vi "PID_controller_13.vi"() -> ()   [LabVIEW 2011]
uses:
  <vilib>/Analysis/NI_AALPro.lvlib
panel:
  out "P(t)":cluster{dbl, "Value":dbl}[](array[cluster])
  in  "Fitting points":i32
  in  "stop":bool
  out "fit":cluster{"element":dbl, "Value":dbl}[](array[cluster])
  out "err_avg":dbl
  out "Setpoint":string
  out "Angle (deg)":string
  in  "Ks":dbl
  out "dt(s)":dbl
  out "windup error":dbl
  out "tPrev":dbl
  out "target value":dbl
  out "error(t-t0)":cluster{dbl, "Value":dbl}[](array[cluster])
  out "error":dbl
  out "tStart(s)":dbl
  out "S00":dbl
  out "S10":dbl
  out "S20":dbl
  out "S11":dbl
  out "S01":dbl
  out "weight":dbl[](array[numeric])
  in  "# of points to watch":i32
  in  "tSmooth(s)":dbl=-1.0
  out "t0":dbl
  out "error(t)":cluster{dbl, "Value":dbl}[](array[cluster])
  out "error out":errorcluster
  out "first":bool=TRUE
  out "P (torr)":string
  out "XY Graph":T1(graph)
  out "current value":dbl
  in  "Period (s)":dbl
  out "dValue":dbl
  out "derivative":dbl
  out "integral":dbl
  out "Current angle (deg)":dbl
  in  "Kd":dbl
  in  "Ki":dbl
  in  "Kp":dbl
  out "Current P (torr)":dbl
  in  "Set Point (torr)":dbl
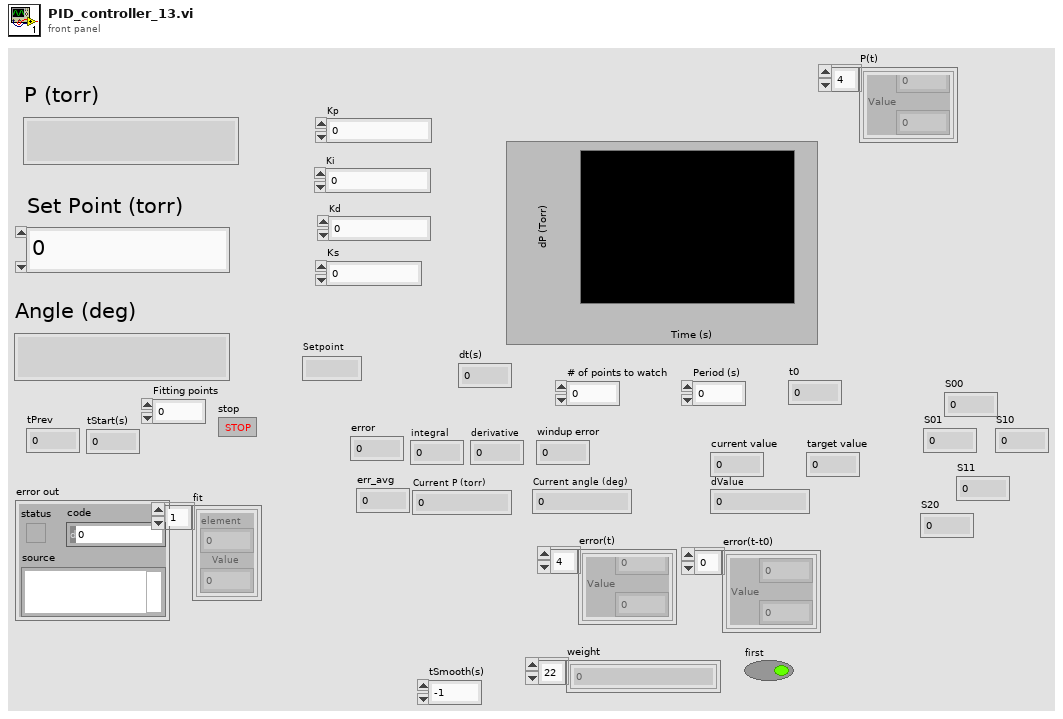
[diagram p1: front panel]
types:
  T1 = cluster{"Value":cluster{"element":dbl, "Value":dbl}[]}[]
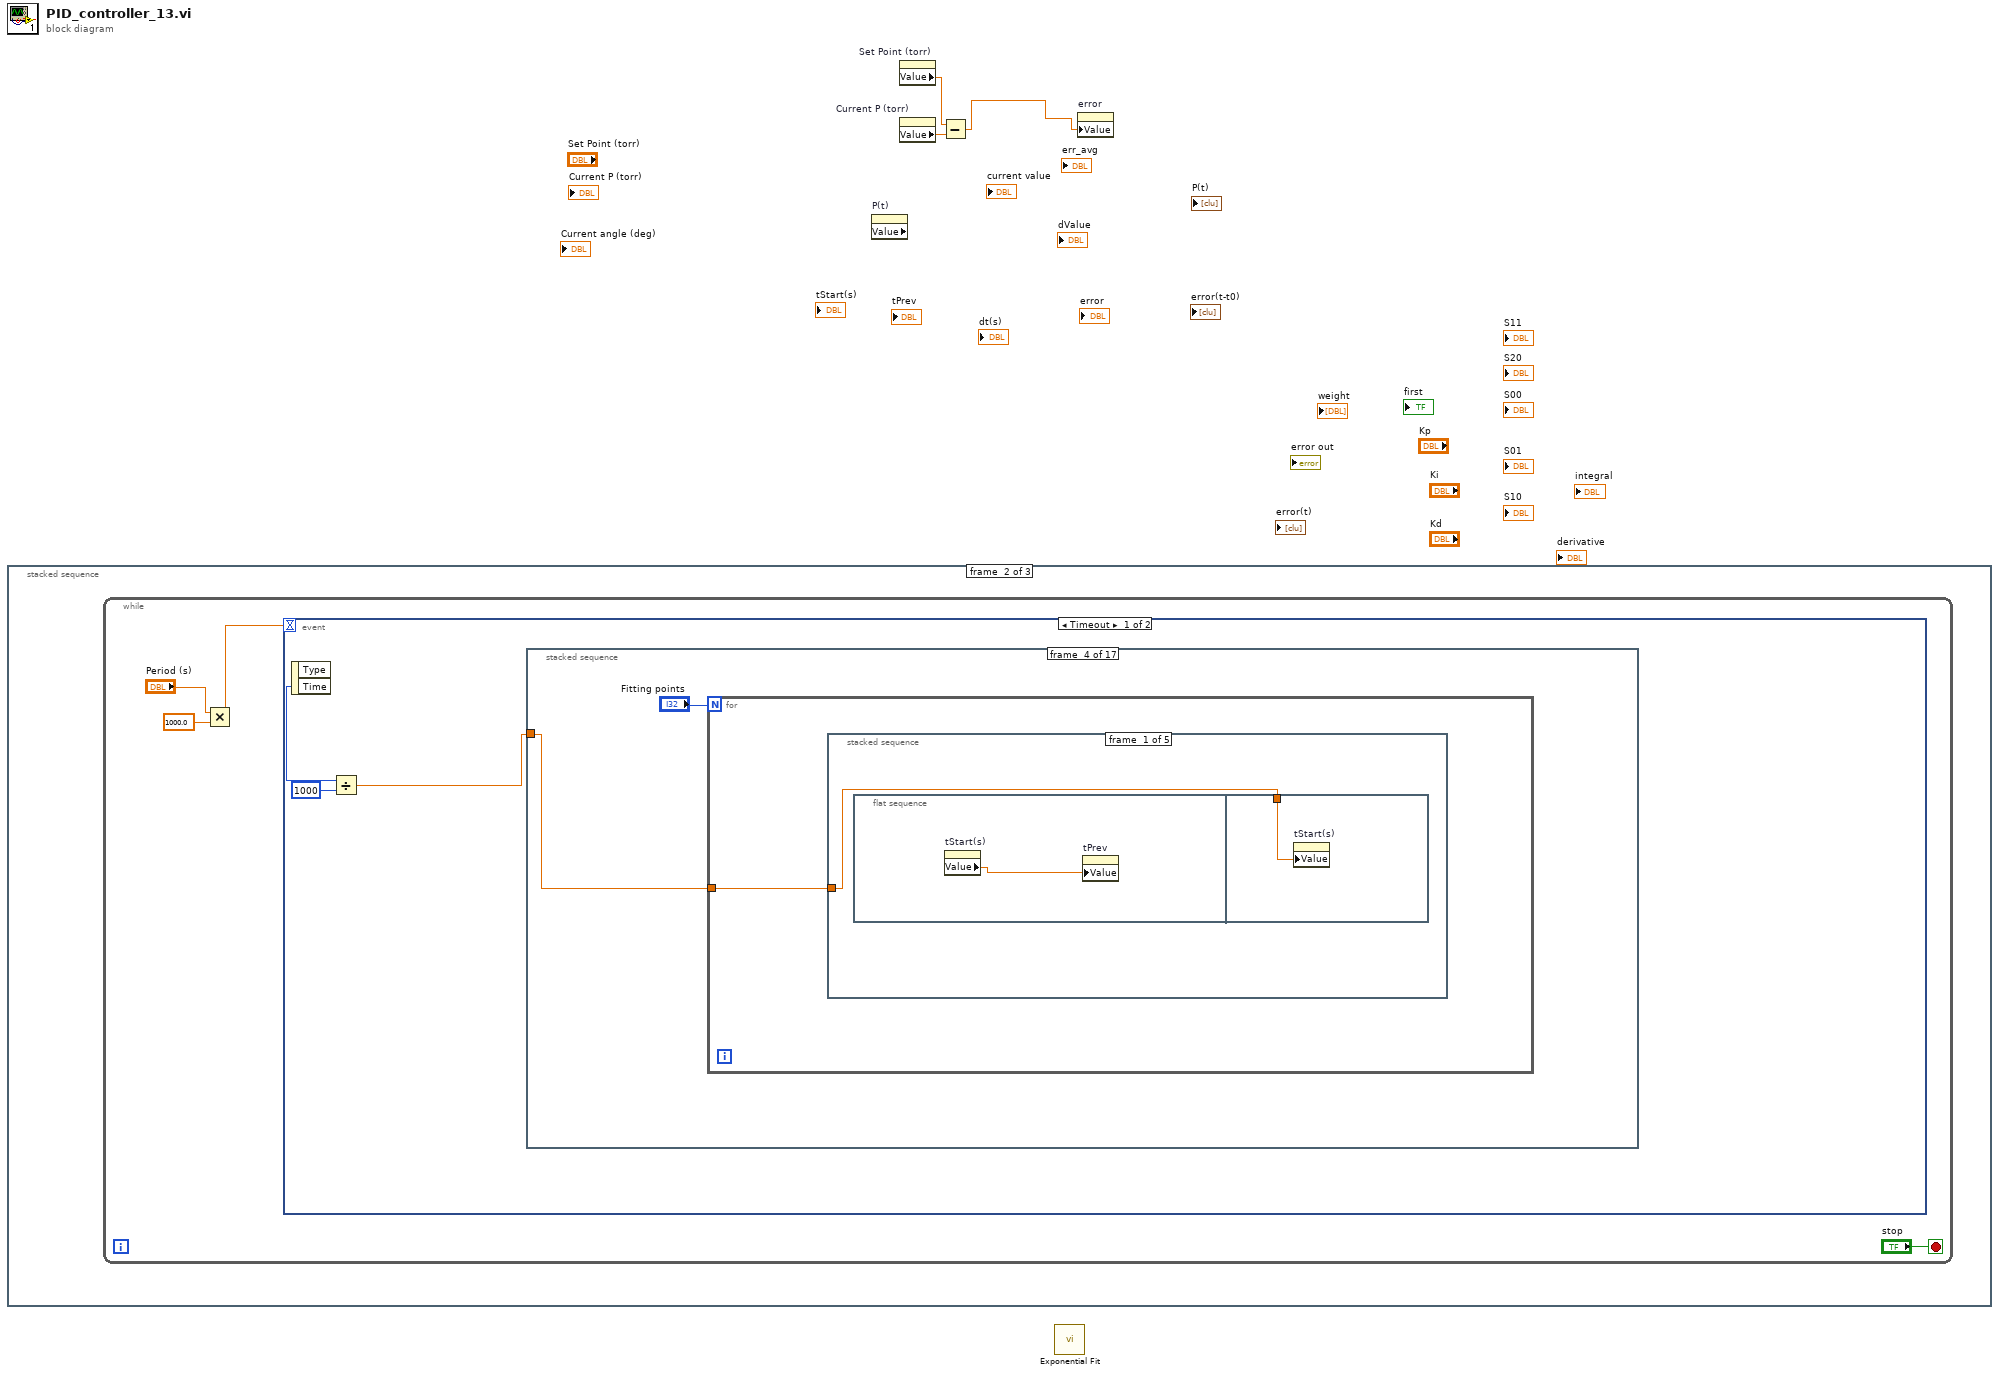
[diagram p0: block diagram]
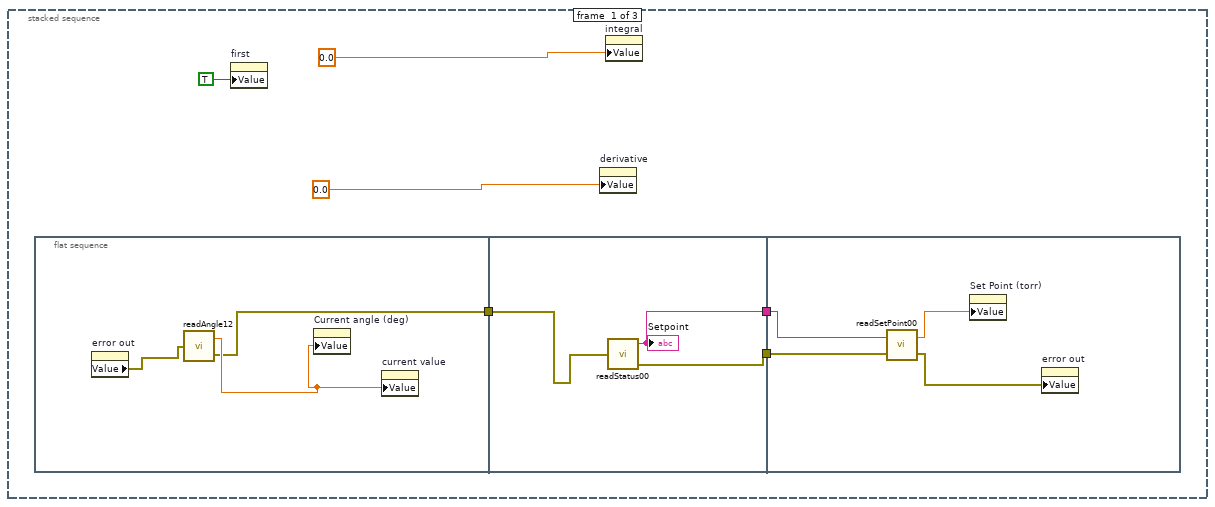
[diagram p2: hidden frame]
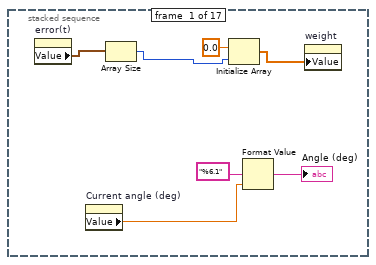
[diagram p3: hidden frame]
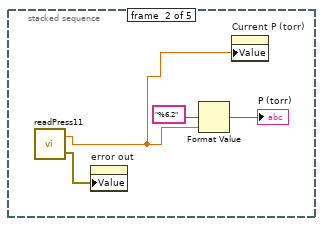
[diagram p6: hidden frame]
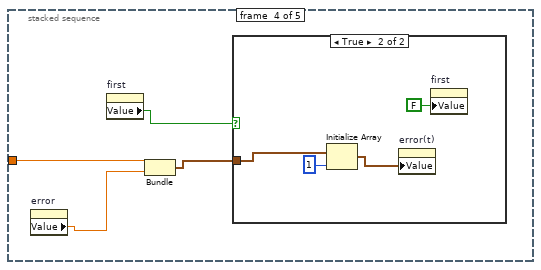
[diagram p8: hidden frame]
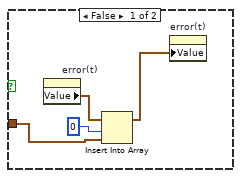
[diagram p9: hidden frame]
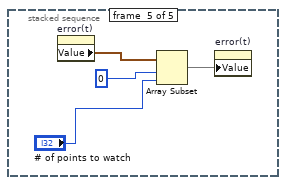
[diagram p10: hidden frame]
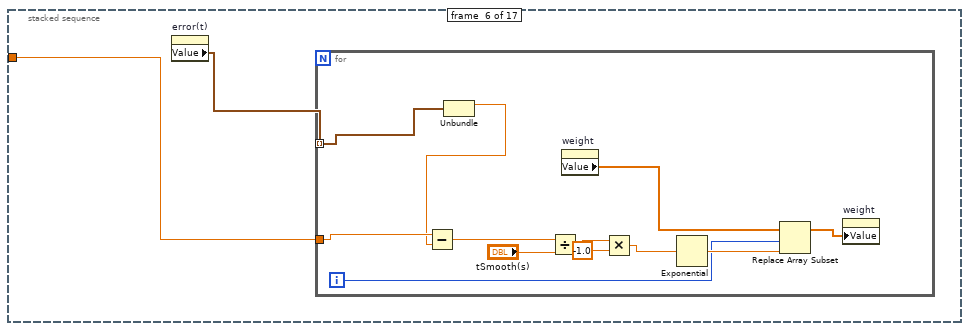
[diagram p12: hidden frame]
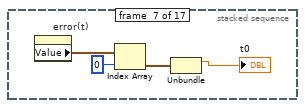
[diagram p13: hidden frame]
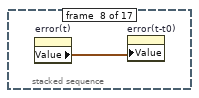
[diagram p14: hidden frame]
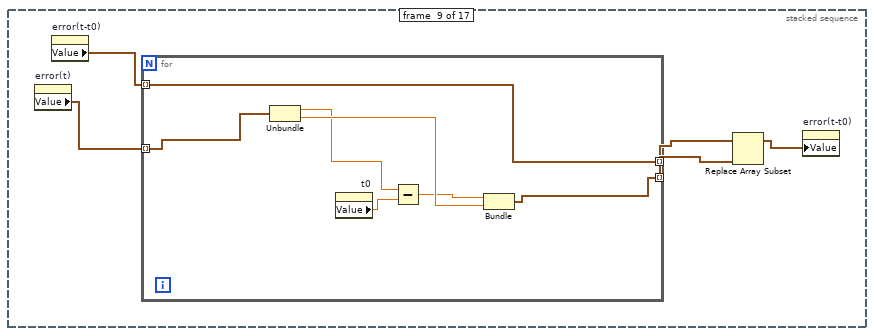
[diagram p15: hidden frame]
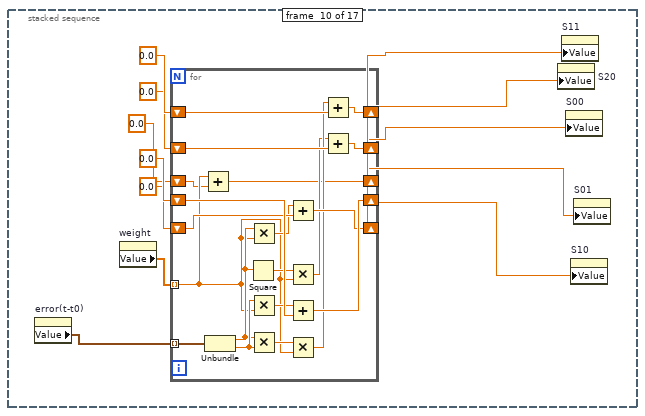
[diagram p16: hidden frame]
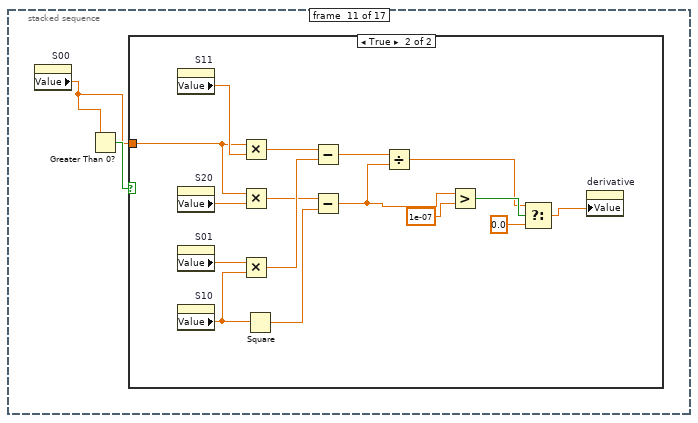
[diagram p17: hidden frame]
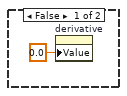
[diagram p18: hidden frame]
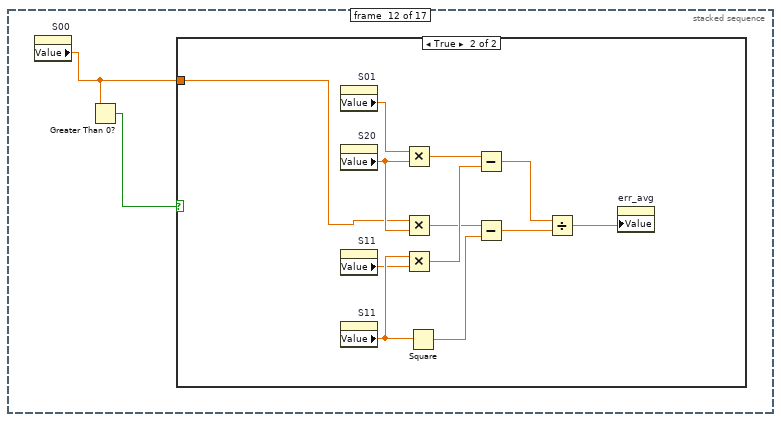
[diagram p19: hidden frame]
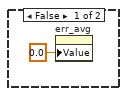
[diagram p20: hidden frame]
diagram:
  n1 = stacked-sequence {
    frame #0 {
      n2 = flat-sequence {
        tunnel: [w10] -> w4
        tunnel: [w15] -> w6
        tunnel: [w14] -> w5
        tunnel: w4 -> [w13]
        tunnel: w6 -> [w19]
        tunnel: w5 -> [w18]
        frame #0 {
          n3 = property on="error out" class="Clust (strict)"() -> ("Value"=w12:errorcluster)  [unwired: 2 in, 2 out]
          n4 = call "readAngle12.vi"("error in"=w12) -> ("angle"=w11:dbl, "error out"=w10:errorcluster)
          n5 = property on="Current angle (deg)" class="DigNum (strict)"("Value"=w11) -> ()  [unwired: 2 in, 2 out]
          n6 = property on="current value" class="DigNum (strict)"("Value"=w11) -> ()  [unwired: 2 in, 2 out]
        }
        frame #1 {
          n7 = call "readStatus00.vi"("error in"=w13) -> ("Setpoint"=w15:string, "error out"=w14:errorcluster)  [unwired: 1 out]
          "Setpoint" <- w15
        }
        frame #2 {
          n8 = call "readSetPoint00.vi"("error in"=w18, "Setpoint"=w19) -> ("error out"=w17:errorcluster, "P"=w16:dbl)
          n9 = property on="Set Point (torr)" class="DigNum (strict)"("Value"=w16) -> ()  [unwired: 2 in, 2 out]
          n10 = property on="error out" class="Clust (strict)"("Value"=w17) -> ()  [unwired: 2 in, 2 out]
        }
      }
      n11 = property on="first" class="Bool (strict)"("Value"=TRUE ("first")) -> ()  [unwired: 2 in, 2 out]
      n12 = property on="derivative" class="DigNum (strict)"("Value"=0.0 ("derivative")) -> ()  [unwired: 2 in, 2 out]
      n13 = property on="integral" class="DigNum (strict)"("Value"=0.0 ("integral")) -> ()  [unwired: 2 in, 2 out]
    }
    frame #1 {
      n14 = while {
        stop <- "stop" stop-if-true
        n15 = Multiply(x="Period (s)", y=1000.0) -> (x*y=w21:dbl)
        n16 = event shown="[0] Timeout" {
          selector: _ -> [_ _]
          dyn-events: _ -> [_ _]
          timeout: w21 -> [_ _]
          event Timeout {
            n17 = event-data() -> ("Time"=w26:u32)  [unwired: 1 in, 1 out]
            n18 = Divide(x=w26, y=u32 1000) -> (x/y=w24:dbl)
            n19 = stacked-sequence {
              tunnel: w24 -> [_ _ w34 w35 _ w61 _ _ _ _ _ _ _ _ _ _ _]
              frame #0 {
                n20 = property on="error(t)" class="Arr (strict)"() -> ("Value"=w30:cluster{dbl, "Value":dbl}[])  [unwired: 2 in, 2 out]
                n21 = property on="Current angle (deg)" class="DigNum (strict)"() -> ("Value"=w31:dbl)  [unwired: 2 in, 2 out]
                n22 = Array Size(array=w30) -> (size(s)=w28:i32)
                n23 = Initialize Array(0.0 ("element"), w28) -> (w27:dbl[])
                n24 = Format Value(format string="%6.1", value (0)=w31) -> (output string=→"Angle (deg)":string)  [unwired: 1 in]
                n25 = property on="weight" class="Arr (strict)"("Value"=w27) -> ()  [unwired: 2 in, 2 out]
              }
              frame #1 {
              }
              frame #2 {
                n26 = stacked-sequence {
                  tunnel: w34 -> [_]
                  frame #0 {
                  }
                }
              }
              frame #3 {
                n27 = for {
                  N: "Fitting points" -> [_]
                  tunnel: w35 -> [w37]
                  n28 = stacked-sequence {
                    tunnel: w37 -> [w38 _ _ w47 _]
                    frame #0 {
                      n29 = flat-sequence {
                        tunnel: w38 -> [w40]
                        frame #0 {
                          n30 = property on="tStart(s)" class="DigNum (strict)"() -> ("Value"=w39:dbl)  [unwired: 2 in, 2 out]
                          n31 = property on="tPrev" class="DigNum (strict)"("Value"=w39) -> ()  [unwired: 2 in, 2 out]
                        }
                        frame #1 {
                          n32 = property on="tStart(s)" class="DigNum (strict)"("Value"=w40) -> ()  [unwired: 2 in, 2 out]
                        }
                      }
                    }
                    frame #1 {
                      n33 = call "readPress11.vi"() -> ("P"=w42:dbl, "error out"=w41:errorcluster)  [unwired: 1 in]
                      n34 = property on="error out" class="Clust (strict)"("Value"=w41) -> ()  [unwired: 2 in, 2 out]
                      n35 = Format Value(format string="%6.2", value (0)=w42) -> (output string=→"P (torr)":string)  [unwired: 1 in]
                      n36 = property on="Current P (torr)" class="DigNum (strict)"("Value"=w42) -> ()  [unwired: 2 in, 2 out]
                    }
                    frame #2 {
                    }
                    frame #3 {
                      n37 = property on="error" class="DigNum (strict)"() -> ("Value"=w45:dbl)  [unwired: 2 in, 2 out]
                      n38 = property on="first" class="Bool (strict)"() -> ("Value"=w48:bool)  [unwired: 2 in, 2 out]
                      n39 = Bundle(w47, "Value"=w45) -> (w46:cluster{dbl, "Value":dbl})  [unwired: 1 in]
                      n40 = case shown="True" w48 {
                        tunnel: w46 -> [w50 w55]
                        frame False {
                          n41 = property on="error(t)" class="Arr (strict)"() -> ("Value"=w51:cluster{dbl, "Value":dbl}[])  [unwired: 2 in, 2 out]
                          n42 = Insert Into Array(array=w51, index=0, new element=w50) -> (w49:cluster{dbl, "Value":dbl}[])
                          n43 = property on="error(t)" class="Arr (strict)"("Value"=w49) -> ()  [unwired: 2 in, 2 out]
                        }
                        frame True {
                          n44 = Initialize Array(w55, 1 ("dimension size")) -> (w53:cluster{dbl, "Value":dbl}[])
                          n45 = property on="error(t)" class="Arr (strict)"("Value"=w53) -> ()  [unwired: 2 in, 2 out]
                          n46 = property on="first" class="Bool (strict)"("Value"=FALSE ("first")) -> ()  [unwired: 2 in, 2 out]
                        }
                      }
                    }
                    frame #4 {
                      n47 = property on="error(t)" class="Arr (strict)"() -> ("Value"=w58:cluster{dbl, "Value":dbl}[])  [unwired: 2 in, 2 out]
                      n48 = Array Subset(array=w58, index=0, length="# of points to watch") -> (w60:cluster{dbl, "Value":dbl}[])
                      n49 = property on="error(t)" class="Arr (strict)"("Value"=w60) -> ()  [unwired: 2 in, 2 out]
                    }
                  }
                }
              }
              frame #4 {
              }
              frame #5 {
                n50 = property on="error(t)" class="Arr (strict)"() -> ("Value"=w62:cluster{dbl, "Value":dbl}[])  [unwired: 2 in, 2 out]
                n51 = for {
                  tunnel: w62 -> [w74] mode=indexing
                  tunnel: w61 -> [w73]
                  i -> [w69]
                  n52 = Unbundle(w74) -> (w72:dbl)  [unwired: 1 out]
                  n53 = Subtract(x=w73, y=w72) -> (x-y=w67:dbl)
                  n54 = Divide(x=w67, y="tSmooth(s)") -> (x/y=w65:dbl)
                  n55 = property on="weight" class="Arr (strict)"() -> ("Value"=w70:dbl[])  [unwired: 2 in, 2 out]
                  n56 = Multiply(x=w65, y=-1.0) -> (x*y=w63:dbl)
                  n57 = Exponential(1:w63) -> (0:w71:dbl)
                  n58 = Replace Array Subset(array=w70, new element=w71, index=w69) -> (w68:dbl[])
                  n59 = property on="weight" class="Arr (strict)"("Value"=w68) -> ()  [unwired: 2 in, 2 out]
                }
              }
              frame #6 {
                n60 = property on="error(t)" class="Arr (strict)"() -> ("Value"=w78:cluster{dbl, "Value":dbl}[])  [unwired: 2 in, 2 out]
                n61 = Index Array(array=w78, index=0) -> (element=w76:cluster{dbl, "Value":dbl})
                n62 = Unbundle(w76) -> (→"t0":dbl)  [unwired: 1 out]
              }
              frame #7 {
                n63 = property on="error(t)" class="Arr (strict)"() -> ("Value"=w79:cluster{dbl, "Value":dbl}[])  [unwired: 2 in, 2 out]
                n64 = property on="error(t-t0)" class="Arr (strict)"("Value"=w79) -> ()  [unwired: 2 in, 2 out]
              }
              frame #8 {
                n65 = property on="error(t)" class="Arr (strict)"() -> ("Value"=w84:cluster{dbl, "Value":dbl}[])  [unwired: 2 in, 2 out]
                n66 = property on="error(t-t0)" class="Arr (strict)"() -> ("Value"=w82:cluster{dbl, "Value":dbl}[])  [unwired: 2 in, 2 out]
                n67 = for {
                  tunnel: w84 -> [w87] mode=indexing
                  tunnel: [w86] -> w83 mode=indexing
                  tunnel: w82 -> [w85] mode=indexing
                  tunnel: [w85] -> w81 mode=indexing
                  n68 = Unbundle(w87) -> (w88:dbl, "Value"=w90:dbl)
                  n69 = property on="t0" class="DigNum (strict)"() -> ("Value"=w91:dbl)  [unwired: 2 in, 2 out]
                  n70 = Subtract(x=w88, y=w91) -> (x-y=w89:dbl)
                  n71 = Bundle(w89, "Value"=w90) -> (w86:cluster{dbl, "Value":dbl})  [unwired: 1 in]
                }
                n72 = Replace Array Subset(array=w81, new element=w83) -> (w80:cluster{dbl, "Value":dbl}[])  [unwired: 1 in]
                n73 = property on="error(t-t0)" class="Arr (strict)"("Value"=w80) -> ()  [unwired: 2 in, 2 out]
              }
              frame #9 {
                n74 = property on="error(t-t0)" class="Arr (strict)"() -> ("Value"=w92:cluster{dbl, "Value":dbl}[])  [unwired: 2 in, 2 out]
                n75 = property on="weight" class="Arr (strict)"() -> ("Value"=w99:dbl[])  [unwired: 2 in, 2 out]
                n76 = for {
                  tunnel: w92 -> [w119] mode=indexing
                  shift-right: [w120] -> w94
                  shift-left: 0.0 -> [w123]
                  shift-right: [w116] -> w97
                  shift-left: 0.0 -> [w122]
                  shift-right: [w115] -> w96
                  shift-left: 0.0 -> [w121]
                  shift-right: [w117] -> w93
                  shift-left: 0.0 -> [w118]
                  tunnel: w99 -> [w106] mode=indexing
                  shift-right: [w104] -> w95
                  shift-left: 0.0 -> [w105]
                  n77 = Add(x=w106, y=w105) -> (x+y=w104:dbl)
                  n78 = Unbundle(w119) -> (w108:dbl, "Value"=w114:dbl)
                  n79 = Square(x=w108) -> (x^2=w110:dbl)
                  n80 = Multiply(x=w108, y=w106) -> (x*y=w107:dbl)
                  n81 = Multiply(x=w114, y=w106) -> (x*y=w113:dbl)
                  n82 = Multiply(x=w108, y=w114) -> (x*y=w112:dbl)
                  n83 = Add(x=w107, y=w118) -> (x+y=w117:dbl)
                  n84 = Multiply(x=w110, y=w106) -> (x*y=w109:dbl)
                  n85 = Add(x=w113, y=w123) -> (x+y=w120:dbl)
                  n86 = Multiply(x=w112, y=w106) -> (x*y=w111:dbl)
                  n87 = Add(x=w111, y=w122) -> (x+y=w116:dbl)
                  n88 = Add(x=w109, y=w121) -> (x+y=w115:dbl)
                }
                n89 = property on="S20" class="DigNum (strict)"("Value"=w96) -> ()  [unwired: 2 in, 2 out]
                n90 = property on="S11" class="DigNum (strict)"("Value"=w97) -> ()  [unwired: 2 in, 2 out]
                n91 = property on="S00" class="DigNum (strict)"("Value"=w95) -> ()  [unwired: 2 in, 2 out]
                n92 = property on="S10" class="DigNum (strict)"("Value"=w93) -> ()  [unwired: 2 in, 2 out]
                n93 = property on="S01" class="DigNum (strict)"("Value"=w94) -> ()  [unwired: 2 in, 2 out]
              }
              frame #10 {
                n94 = property on="S00" class="DigNum (strict)"() -> ("Value"=w124:dbl)  [unwired: 2 in, 2 out]
                n95 = Greater Than 0?(x=w124) -> (x > 0?=w125:bool)
                n96 = case shown="True" w125 {
                  tunnel: w124 -> [_ w134]
                  frame False {
                    n97 = property on="derivative" class="DigNum (strict)"("Value"=0.0 ("derivative")) -> ()  [unwired: 2 in, 2 out]
                  }
                  frame True {
                    n98 = property on="S11" class="DigNum (strict)"() -> ("Value"=w136:dbl)  [unwired: 2 in, 2 out]
                    n99 = property on="S20" class="DigNum (strict)"() -> ("Value"=w135:dbl)  [unwired: 2 in, 2 out]
                    n100 = property on="S01" class="DigNum (strict)"() -> ("Value"=w133:dbl)  [unwired: 2 in, 2 out]
                    n101 = property on="S10" class="DigNum (strict)"() -> ("Value"=w137:dbl)  [unwired: 2 in, 2 out]
                    n102 = Multiply(x=w134, y=w136) -> (x*y=w142:dbl)
                    n103 = Multiply(x=w134, y=w135) -> (x*y=w140:dbl)
                    n104 = Multiply(x=w133, y=w137) -> (x*y=w141:dbl)
                    n105 = Square(x=w137) -> (x^2=w139:dbl)
                    n106 = Subtract(x=w142, y=w141) -> (x-y=w138:dbl)
                    n107 = Subtract(x=w140, y=w139) -> (x-y=w132:dbl)
                    n108 = Divide(x=w138, y=w132) -> (x/y=w128:dbl)
                    n109 = Greater?(x=w132, y=1e-07) -> (0:w130:bool)
                    n110 = Select(t=w128, s=w130, f=0.0) -> (s? t:f=w129:dbl)
                    n111 = property on="derivative" class="DigNum (strict)"("Value"=w129) -> ()  [unwired: 2 in, 2 out]
                  }
                }
              }
              frame #11 {
                n112 = property on="S00" class="DigNum (strict)"() -> ("Value"=w143:dbl)  [unwired: 2 in, 2 out]
                n113 = Greater Than 0?(x=w143) -> (x > 0?=w144:bool)
                n114 = case shown="True" w144 {
                  tunnel: w143 -> [_ w147]
                  frame False {
                    n115 = property on="err_avg" class="DigNum (strict)"("Value"=0.0 ("Pavg")) -> ()  [unwired: 2 in, 2 out]
                  }
                  frame True {
                    n116 = property on="S01" class="DigNum (strict)"() -> ("Value"=w148:dbl)  [unwired: 2 in, 2 out]
                    n117 = property on="S20" class="DigNum (strict)"() -> ("Value"=w151:dbl)  [unwired: 2 in, 2 out]
                    n118 = property on="S11" class="DigNum (strict)"() -> ("Value"=w149:dbl)  [unwired: 2 in, 2 out]
                    n119 = property on="S11" class="DigNum (strict)"() -> ("Value"=w150:dbl)  [unwired: 2 in, 2 out]
                    n120 = Multiply(x=w148, y=w151) -> (x*y=w156:dbl)
                    n121 = Multiply(x=w147, y=w151) -> (x*y=w153:dbl)
                    n122 = Multiply(x=w150, y=w149) -> (x*y=w157:dbl)
                    n123 = Square(x=w150) -> (x^2=w154:dbl)
                    n124 = Subtract(x=w156, y=w157) -> (x-y=w152:dbl)
                    n125 = Subtract(x=w153, y=w154) -> (x-y=w155:dbl)
                    n126 = Divide(x=w152, y=w155) -> (x/y=w146:dbl)
                    n127 = property on="err_avg" class="DigNum (strict)"("Value"=w146) -> ()  [unwired: 2 in, 2 out]
                  }
                }
              }
              frame #12 {
                n128 = property on="error(t-t0)" class="Arr (strict)"() -> ("Value"=w161:cluster{dbl, "Value":dbl}[])  [unwired: 2 in, 2 out]
                n129 = Array Size(array=w161) -> (size(s)=w160:i32)
                n130 = Greater?(x=w160, y=1) -> (0:w158:bool)
                n131 = case shown="True" w158 {
                  frame False {
                  }
                  frame True {
                    n132 = property on="error(t-t0)" class="Arr (strict)"() -> ("Value"=w165:cluster{dbl, "Value":dbl}[])  [unwired: 2 in, 2 out]
                    n133 = Array Size(array=w165) -> (size(s)=w175:i32)
                    n134 = Index Array(array=w165, index=0) -> (element=w173:cluster{dbl, "Value":dbl})
                    n135 = Unbundle(w173) -> (w168:dbl)  [unwired: 1 out]
                    n136 = Decrement(x=w175) -> (x-1=w174:i32)
                    n137 = Index Array(array=w165, index=w174) -> (element=w172:cluster{dbl, "Value":dbl})
                    n138 = Unbundle(w172) -> (w166:dbl)  [unwired: 1 out]
                    n139 = property on="derivative" class="DigNum (strict)"() -> ("Value"=w171:dbl)  [unwired: 2 in, 2 out]
                    n140 = property on="error" class="DigNum (strict)"() -> ("Value"=w169:dbl)  [unwired: 2 in, 2 out]
                    n141 = Multiply(x=w166, y=w171) -> (x*y=w170:dbl)
                    n142 = Add(x=w169, y=w170) -> (x+y=w167:dbl)
                    n143 = Bundle(w168, "Value"=w169) -> (w164:cluster{dbl, "Value":dbl})  [unwired: 1 in]
                    n144 = Bundle(w166, w167) -> (w163:cluster{dbl, dbl})  [unwired: 1 in]
                    n145 = Build Array(w164, w163) -> (→"fit":cluster{dbl, "Value":dbl}[])
                  }
                }
              }
              frame #13 {
                n146 = property on="error" class="DigNum (strict)"() -> ("Value"=w181:dbl)  [unwired: 2 in, 2 out]
                n147 = property on="tPrev" class="DigNum (strict)"() -> ("Value"=w182:dbl)  [unwired: 2 in, 2 out]
                n148 = property on="tStart(s)" class="DigNum (strict)"() -> ("Value"=w183:dbl)  [unwired: 2 in, 2 out]
                n149 = Subtract(x=w183, y=w182) -> (x-y=w177:dbl)
                n150 = property on="dt(s)" class="DigNum (strict)"("Value"=w177) -> ()  [unwired: 2 in, 2 out]
                n151 = property on="integral" class="DigNum (strict)"() -> ("Value"=w179:dbl)  [unwired: 2 in, 2 out]
                n152 = Multiply(x=w181, y=w177) -> (x*y=w180:dbl)
                n153 = Add(x=w180, y=w179) -> (x+y=w178:dbl)
                n154 = property on="integral" class="DigNum (strict)"("Value"=w178) -> ()  [unwired: 2 in, 2 out]
              }
              frame #14 {
                n155 = property on="error" class="DigNum (strict)"() -> ("Value"=w184:dbl)  [unwired: 2 in, 2 out]
                n156 = property on="Kp" class="DigNum (strict)"() -> ("Value"=w194:dbl)  [unwired: 2 in, 2 out]
                n157 = property on="integral" class="DigNum (strict)"() -> ("Value"=w192:dbl)  [unwired: 2 in, 2 out]
                n158 = property on="derivative" class="DigNum (strict)"() -> ("Value"=w190:dbl)  [unwired: 2 in, 2 out]
                n159 = property on="Ki" class="DigNum (strict)"() -> ("Value"=w193:dbl)  [unwired: 2 in, 2 out]
                n160 = property on="Kd" class="DigNum (strict)"() -> ("Value"=w191:dbl)  [unwired: 2 in, 2 out]
                n161 = Multiply(x=w191, y=w190) -> (x*y=w187:dbl)
                n162 = Multiply(x=w193, y=w192) -> (x*y=w188:dbl)
                n163 = Multiply(x=w194, y=w184) -> (x*y=w189:dbl)
                n164 = Add(x=w189, y=w188) -> (x+y=w186:dbl)
                n165 = Add(x=w186, y=w187) -> (x+y=w185:dbl)
                n166 = property on="dValue" class="DigNum (strict)"("Value"=w185) -> ()  [unwired: 2 in, 2 out]
              }
              frame #15 {
                w204 = 90.0 ("y")
                n167 = property on="dValue" class="DigNum (strict)"() -> ("Value"=w211:dbl)  [unwired: 2 in, 2 out]
                n168 = property on="current value" class="DigNum (strict)"() -> ("Value"=w212:dbl)  [unwired: 2 in, 2 out]
                n169 = Add(x=w212, y=w211) -> (x+y=w195:dbl)
                "target value" <- w195
                n170 = Less Than 0?(x=w195) -> (x < 0?=w208:bool)
                n171 = Select(t=0.0, s=w208, f=w195) -> (s? t:f=w205:dbl)
                n172 = property on="error out" class="Clust (strict)"() -> ("Value"=w210:errorcluster)  [unwired: 2 in, 2 out]
                n173 = Greater?(x=w205, y=w204) -> (0:w206:bool)
                n174 = Select(t=w204, s=w206, f=w205) -> (s? t:f=w196:dbl)
                n175 = Subtract(x=w196, y=w195) -> (x-y=w203:dbl)
                "windup error" <- w203
                n176 = call "setAngle_00.vi"("error in (no error)"=w210, "Angle (deg)"=w196) -> ("error out"=w209:errorcluster)
                n177 = property on="Current angle (deg)" class="DigNum (strict)"("Value"=w196) -> ()  [unwired: 2 in, 2 out]
                n178 = property on="dt(s)" class="DigNum (strict)"() -> ("Value"=w202:dbl)  [unwired: 2 in, 2 out]
                n179 = property on="current value" class="DigNum (strict)"("Value"=w196) -> ()  [unwired: 2 in, 2 out]
                n180 = property on="error out" class="Clust (strict)"("Value"=w209) -> ()  [unwired: 2 in, 2 out]
                n181 = Multiply(x=w203, y=w202) -> (x*y=w201:dbl)
                n182 = property on="integral" class="DigNum (strict)"() -> ("Value"=w198:dbl)  [unwired: 2 in, 2 out]
                n183 = Multiply(x="Ks", y=w201) -> (x*y=w199:dbl)
                n184 = Add(x=w199, y=w198) -> (x+y=w197:dbl)
                n185 = property on="integral" class="DigNum (strict)"("Value"=w197) -> ()  [unwired: 2 in, 2 out]
              }
              frame #16 {
                n186 = property on="fit" class="Arr (strict)"() -> ("Value"=w215:cluster{"element":dbl, "Value":dbl}[])  [unwired: 2 in, 2 out]
                n187 = property on="error(t-t0)" class="Arr (strict)"() -> ("Value"=w214:cluster{dbl, "Value":dbl}[])  [unwired: 2 in, 2 out]
                n188 = Build Cluster Array(w214, w215) -> (→"XY Graph":T1)
              }
            }
          }
          event "Set Point (torr)": Value Change {
            n189 = event-data() -> ()  [unwired: 1 in, 5 out]
            n190 = property on="Set Point (torr)" class="DigNum (strict)"() -> ("Value"=w218:dbl)  [unwired: 2 in, 2 out]
            n191 = property on="Setpoint" class="Str"() -> ("Value"=w219:string)  [unwired: 2 in, 2 out]
            n192 = property on="error out" class="Clust (strict)"() -> ("Value"=w217:errorcluster)  [unwired: 2 in, 2 out]
            n193 = call "writeSetPoint_00.vi"("error in"=w217, "P (Torr)"=w218, "Setpoint"=w219) -> ("error out"=w216:errorcluster)
            n194 = property on="error out" class="Clust (strict)"("Value"=w216) -> ()  [unwired: 2 in, 2 out]
          }
        }
      }
    }
    frame #2 {
      n195 = flat-sequence {
        frame #0 {
          n196 = call "WriteAdaptorr03.vi"("string to write"="D5") -> ()  [unwired: 1 in, 1 out]
        }
        frame #1 {
          n197 = property on="Setpoint" class="Str"() -> ("Value"=w222:string)  [unwired: 2 in, 2 out]
          n198 = Concatenate Strings("Press ", w222, " on AdapTorr") -> (w221:string)
          n199 = One Button Dialog(message=w221) -> ()  [unwired: 1 in, 1 out]
        }
      }
    }
  }
  n200 = property on="P(t)" class="Arr (strict)" props=["Value"]() -> ()  [unwired: 2 in, 3 out]
  n201 = property on="Set Point (torr)" class="DigNum (strict)"() -> ("Value"=w2:dbl)  [unwired: 2 in, 2 out]
  n202 = property on="Current P (torr)" class="DigNum (strict)"() -> ("Value"=w1:dbl)  [unwired: 2 in, 2 out]
  n203 = Subtract(x=w2, y=w1) -> (x-y=w3:dbl)
  n204 = call <vilib>:"Exponential Fit.vi"() -> ()  [unwired: 10 in, 6 out]
  n205 = property on="error" class="DigNum (strict)"("Value"=w3) -> ()  [unwired: 2 in, 2 out]
